vi "Read Stop Observer Loop.vi"(8 "error in (no error)":errorcluster, 11 "Device Connector in":refnum<class "Device Connector.lvclass">) -> (0 "error out":errorcluster, 2 "Stop Observer Loop":T1, 3 "Device Connector out":refnum<class "Device Connector.lvclass">)   [LabVIEW 2024, in "Device Connector.lvclass"]
uses:
  Device Connector.lvclass
  Type Def/Stop Observer Loop.ctl
  Device Connector.lvclass/Device Connector.ctl
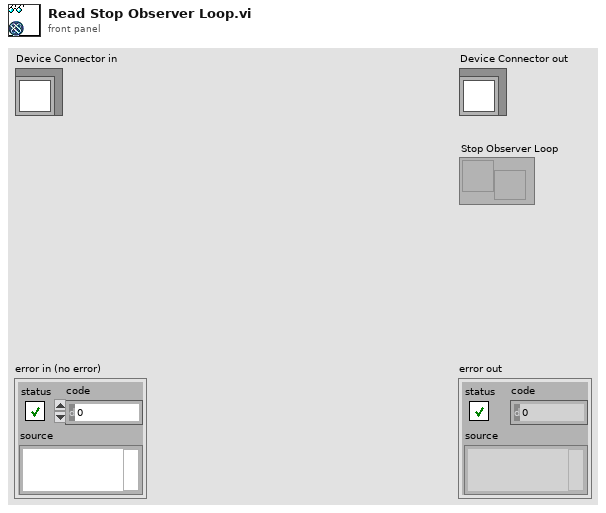
[diagram p1: front panel]
types:
  T1 = typedef "Stop Observer Loop.ctl" = refnum<notifier>
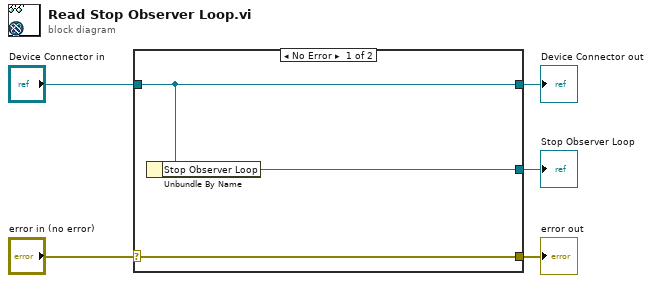
[diagram p0: block diagram]
diagram:
  n1 = case shown="No Error" "error in (no error)" {
    selector: "error in (no error)" -> [w8 w9]
    tunnel: [w8 w9] -> w4
    tunnel: [w7 w10] -> w2
    tunnel: "Device Connector in" -> [w7 w10]
    tunnel: [w6 _] -> w1
    frame No Error {
      n2 = Unbundle By Name(w7) -> ("Stop Observer Loop"=w6:T1)
    }
    frame Error {
    }
  }
  "error out" <- w4
  "Device Connector out" <- w2
  "Stop Observer Loop" <- w1
